vi "TALLER QUIZ CUARTO PUNTO.vi"() -> ()   [LabVIEW 2019]
panel:
  out "BANDA":i64(slide) scale=0.0..1200.0
  in  "DIRECCION":bool
  in  "STAR-STOP":bool
  in  "VELOCIDAD m/300ms":dbl(knob) scale=1.0..10.0
  # "DERECHA"
  # "IZQUIERDA"
  # "POSICION"
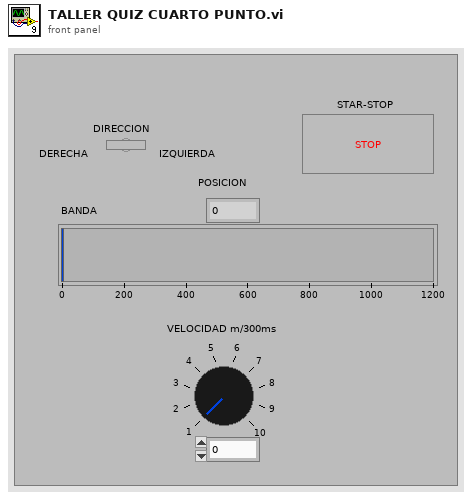
[diagram p1: front panel]
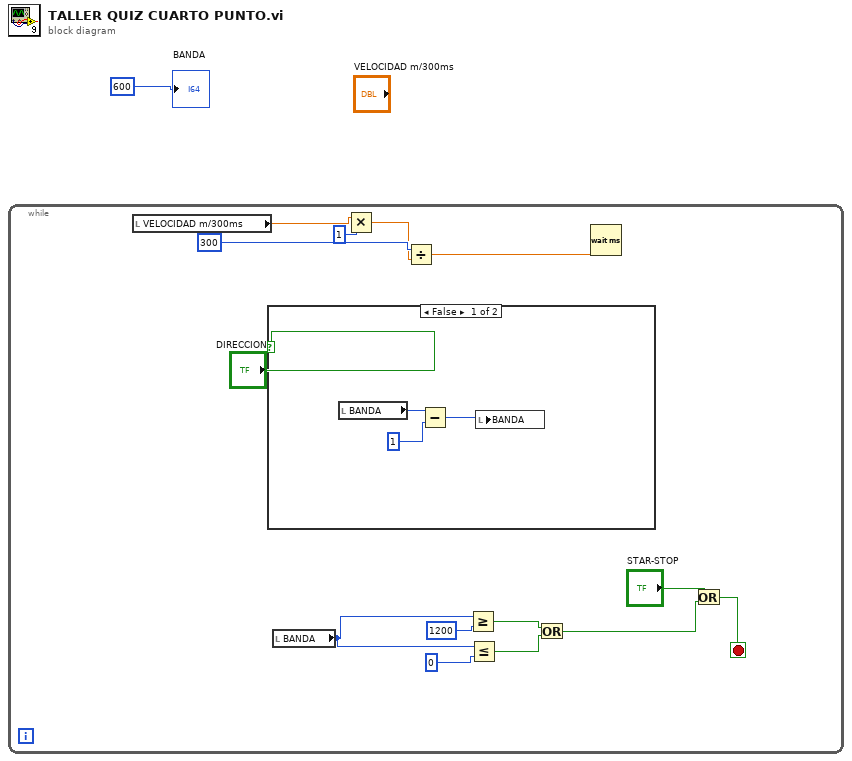
[diagram p0: block diagram]
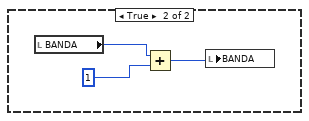
[diagram p2: hidden frame]
diagram:
  n1 = while {
    stop <- w5 stop-if-true
    n2 = local read "VELOCIDAD m/300ms"() -> (w13:dbl)
    n3 = case shown="False" "DIRECCION" {
      frame False {
        n4 = local read "BANDA"() -> (w18:i64)
        n5 = Subtract(x=w18, y=1) -> (x-y=w16:i64)
        n6 = local write "BANDA"(w16) -> ()
      }
      frame True {
        n7 = local read "BANDA"() -> (w21:i64)
        n8 = Add(x=w21, y=1) -> (x+y=w20:i64)
        n9 = local write "BANDA"(w20) -> ()
      }
    }
    n10 = local read "BANDA"() -> (w10:i64)
    n11 = Multiply(x=w13, y=1) -> (x*y=w12:dbl)
    n12 = Divide(x=300, y=w12) -> (x/y=w11:dbl)
    n13 = Greater Or Equal?(x=w10, y=1200) -> (x >= y?=w4:bool)
    n14 = Less Or Equal?(x=w10, y=0) -> (x <= y?=w3:bool)
    n15 = Or(x=w4, y=w3) -> (x .or. y?=w6:bool)
    n16 = Wait (ms)(milliseconds to wait=w11) -> ()  [unwired: 1 out]
    n17 = Or(x="STAR-STOP", y=w6) -> (x .or. y?=w5:bool)
  }
  "BANDA" <- 600
